vi "FTW-Supervisor-Connect.vi"(5 "Supervisor Address":string, 11 "error in":errorcluster) -> (4 "FTW Supervisor Connection":T1, 15 "error out":errorcluster)   [LabVIEW 2015]
uses:
  core/type/FTW-Type-Actor-Connector.ctl
panel:
  # "Inputs"
  # "Outputs"
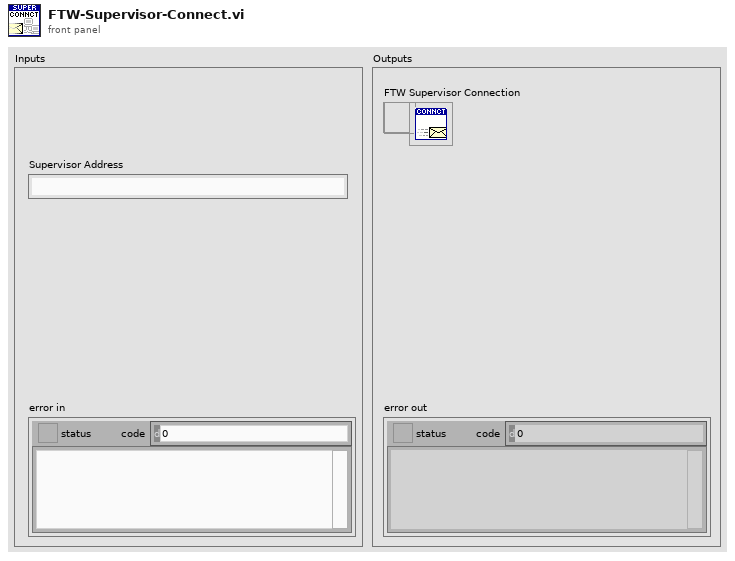
[diagram p1: front panel]
types:
  T1 = typedef "FTW-Type-Actor-Connector.ctl" = refnum<data-value>
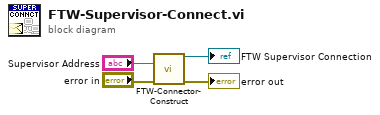
[diagram p0: block diagram]
diagram:
  n1 = call "FTW-Connector-Construct.vi"("Remote Inbox Address"="Supervisor Address", "error in"="error in") -> ("FTW Actor Connector"=→"FTW Supervisor Connection":T1, "error out"=→"error out":errorcluster)  [unwired: 12 in]
